vi "Publish file.vi"(10 "Publish files":string[](array[string]), 11 "filename":string) -> (7 "Yes":bool)   [LabVIEW 2012]
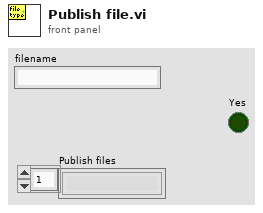
[diagram p1: front panel]
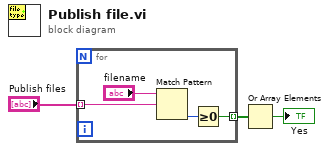
[diagram p0: block diagram]
diagram:
  n1 = for {
    tunnel: "Publish files" -> [w6] mode=indexing
    tunnel: [w4] -> w1 mode=indexing
    n2 = Match Pattern(string="filename", regular expression=w6) -> (offset past match=w5:i32)  [unwired: 1 in, 3 out]
    n3 = Greater Or Equal To 0?(x=w5) -> (x >= 0?=w4:bool)
  }
  n4 = Or Array Elements(Boolean array=w1) -> (logical OR=→"Yes":bool)
